vi "MIU_Control_v1.4 - Working - has bugs still.vi"() -> ()   [LabVIEW 2010]
uses:
  <vilib>/Utility/error.llb/DialogType.ctl
  <vilib>/Instr/_visa.llb/VISA Configure Serial Port (Instr).vi
  <vilib>/Analysis/NI_AALPro.lvlib
panel:
  in  "Tab Control":T1(tab)
  in  "Serial Read Port":refnum<visa-resource-name>="COM5"
  in  "data bits":u16=8 min=5 max=8 step=1
  in  "parity":u16(ring) items=["None", "Odd", "Even", "Mark", "Space"]
  in  "stop bits":u16(ring)=10 items=["1.0"=10, "1.5"=15, "2.0"=20]
  in  "flow control":u16(ring) items=["None"=0, "XON/XOFF"=1, "RTS/CTS"=2, "DTR/DSR"=4]
  in  "delay before read (ms)":u32=500
  in  "byte count":u32=500
  out "Incoming Serial String":string="    02/28/13 05:18:49.492,    3.20644e-01,    0.00000e+00,    3.33105e-01,    0.00000e+00,    5.19723e+02,    0.00000e+00,    3.20811e-01,    0.00000e+00,    3.33278e-01,    0.00000e+00,    8.02680e+01,    0.00000e+00,    3.33389e+01,    0.00000e+00,    2.71783e+01,    0.00000e+00,    3.55973e-01,    0.00000e+00,    6.31022e-01,    0.00000e+00,    1.95007e+00,    0.00000e+00,              3\n"
  out "Time":string="05:18:49.492"
  out "Date":string="02/28/13"
  out "return count":u32=394
  in  "Instrument baud rate (9600)":u32=9600
  in  "Control Port":refnum<visa-resource-name>="COM4"
  in  "Control baud rate":u32=9600
  out "N2O is FLAT":bool
  out "Rolling CO Slope Fit":cluster{i32[], "Best Linear Fit":dbl[]}[](graph)=[{[0, 1, 2, 3, 4, 5, 6, 7, 8, 9, 10, 11, 12, 13, 14, 15, 16, 17, 18, 19], "Best Linear Fit"=[0.320611, 0.320505, 0.320476, 0.3208, 0.320926, 0.320701, 0.320587, 0.320889, 0.320914, 0.320439, 0.3209, 0.320794, 0.320847, 0.320592, 0.320735, 0.32085, 0.320821, 0.320729, 0.320589, 0.320309]}, {[0, 1, 2, 3, 4, 5, 6, 7, 8, 9, 10, 11, 12, 13, 14, 15, 16, 17, 18, 19], "Best Linear Fit"=[0.32070674285714285, 0.3207061067669173, 0.3207054706766917, 0.32070483458646615, 0.3207041984962406, 0.32070356240601505, 0.32070292631578945, 0.3207022902255639, 0.32070165413533835, 0.3207010180451128, 0.3207003819548872, 0.32069974586466166, 0.3206991097744361, 0.32069847368421056, 0.32069783759398496, 0.3206972015037594, 0.32069656541353386, 0.32069592932330826, 0.3206952932330827, 0.32069465714285716]}]
  out "CO":dbl(graph)=0.320644
  out "N2O":dbl(graph)=0.333105
  out "H2O":dbl(graph)=519.723
  out "CO PPM":string=" 3.20644e-01"
  out "N2O PPM":string="3.33105e-01"
  out "H2O PPM":string="5.19723e+02"
  in  "Points to Average":i32=30
  out "CO Slope":dbl=-6.360902255623756e-07
  out "Rolling N2O Slope Fit 2":cluster{i32[], "Best Linear Fit":dbl[]}[](graph)=[{[0, 1, 2, 3, 4, 5, 6, 7, 8, 9, 10, 11, 12, 13, 14, 15, 16, 17, 18, 19], "Best Linear Fit"=[0.333232, 0.332975, 0.333256, 0.333094, 0.333062, 0.3332, 0.332763, 0.333281, 0.333155, 0.333115, 0.333375, 0.33321, 0.333348, 0.33294, 0.333468, 0.333464, 0.333003, 0.333373, 0.33336, 0.333239]}, {[0, 1, 2, 3, 4, 5, 6, 7, 8, 9, 10, 11, 12, 13, 14, 15, 16, 17, 18, 19], "Best Linear Fit"=[0.33308077142857145, 0.33309286390977444, 0.3331049563909775, 0.33311704887218047, 0.3331291413533835, 0.3331412338345865, 0.3331533263157895, 0.3331654187969925, 0.3331775112781955, 0.33318960375939854, 0.33320169624060153, 0.3332137887218045, 0.33322588120300756, 0.33323797368421054, 0.3332500661654135, 0.33326215864661657, 0.33327425112781955, 0.3332863436090226, 0.3332984360902256, 0.33331052857142857]}]
  out "N2O Slope":dbl=1.209248120300707e-05
  in  "N2O Low Limit":dbl=-1e-05
  in  "CO High Limit":dbl=1e-05
  out "CO is FLAT":bool
  in  "CO Low Limit":dbl=-1e-05
  in  "N2O High Limit":dbl=1e-05
  out "Switch Valve":bool
  out "Boolean":bool
  in  "Manually Switch Valves":bool=TRUE
  in  "Valve to switch":dbl=1.0 min=0.0 max=16.0 step=1.0
  in  "stop":bool
  in  "Switching Delay (s)":dbl=60.0
  out "Current Valve":dbl=1.0
  in  "Number of Bottles":dbl=5.0
  out "CELL TEMP":string="3.33389e+01"
  out "CELL TEMPERATURE":dbl(graph)=33.3389
  out "AMBIENT TEMPERATURE":dbl(graph)=27.1783
  out "AMBIENT TEMP":string="2.71783e+01"
  out "AIN5":dbl(graph)=0.631022
  out "SUPERCOOL TEMP":string="6.31022e-01"
  out "LINE LOCK":dbl(graph)=0.355973
  out "LINELOCK - LASER CONTROL VOLTAGE":string="3.55973e-01"
  out "PRESSURE":dbl(graph)=80.268
  out "PRESSURE 2":string="8.02680e+01"
  out "CO DRY 2":dbl(graph)=0.320811
  out "N2O DRY":dbl(graph)=0.333278
  out "CO DRY":string="3.20811e-01"
  out "N2O DRY 2":string="3.33278e-01"
  # "Automatic Linearization"
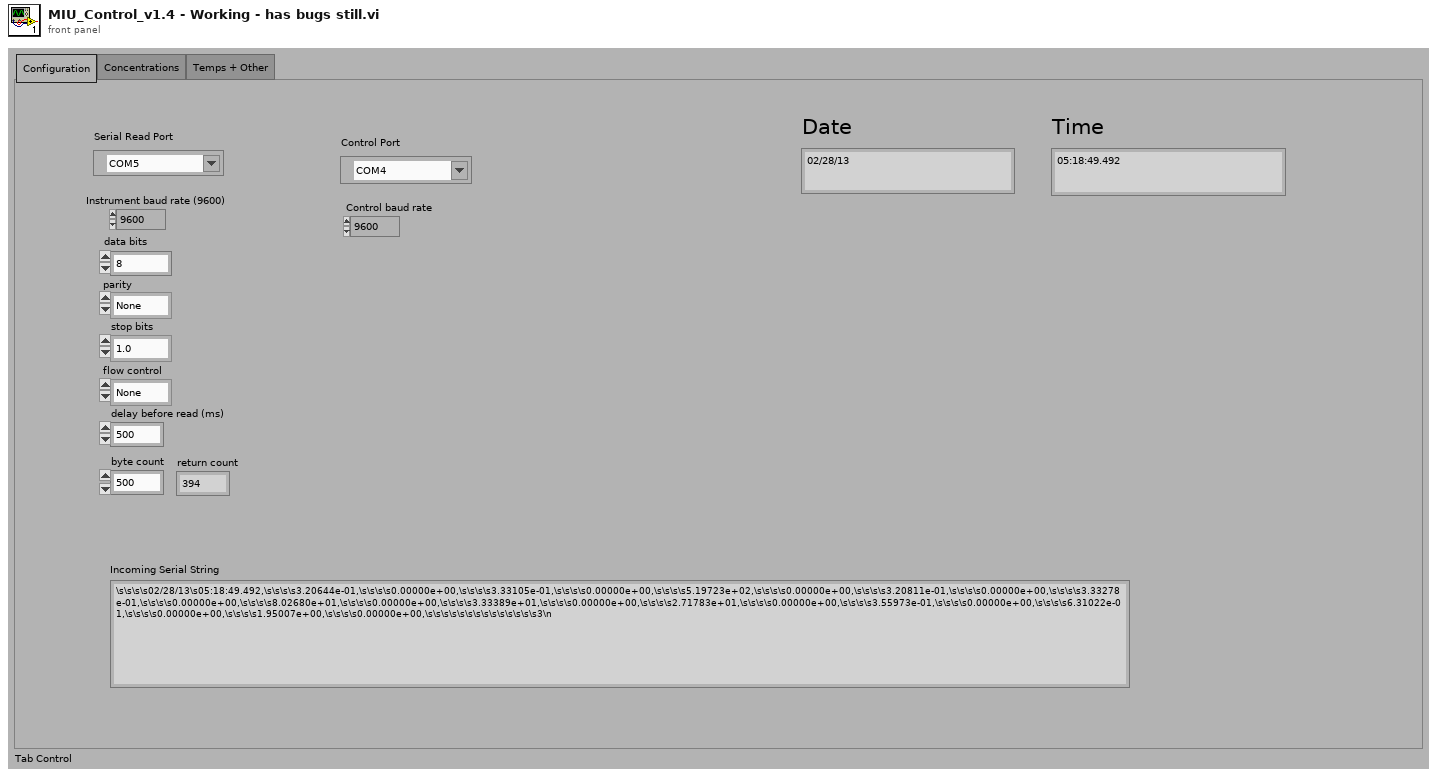
[diagram p1: front panel]
types:
  T1 = enum32{"Configuration", "Concentrations", "Temps + Other"}
  T2 = typedef "DialogType.ctl" = u16
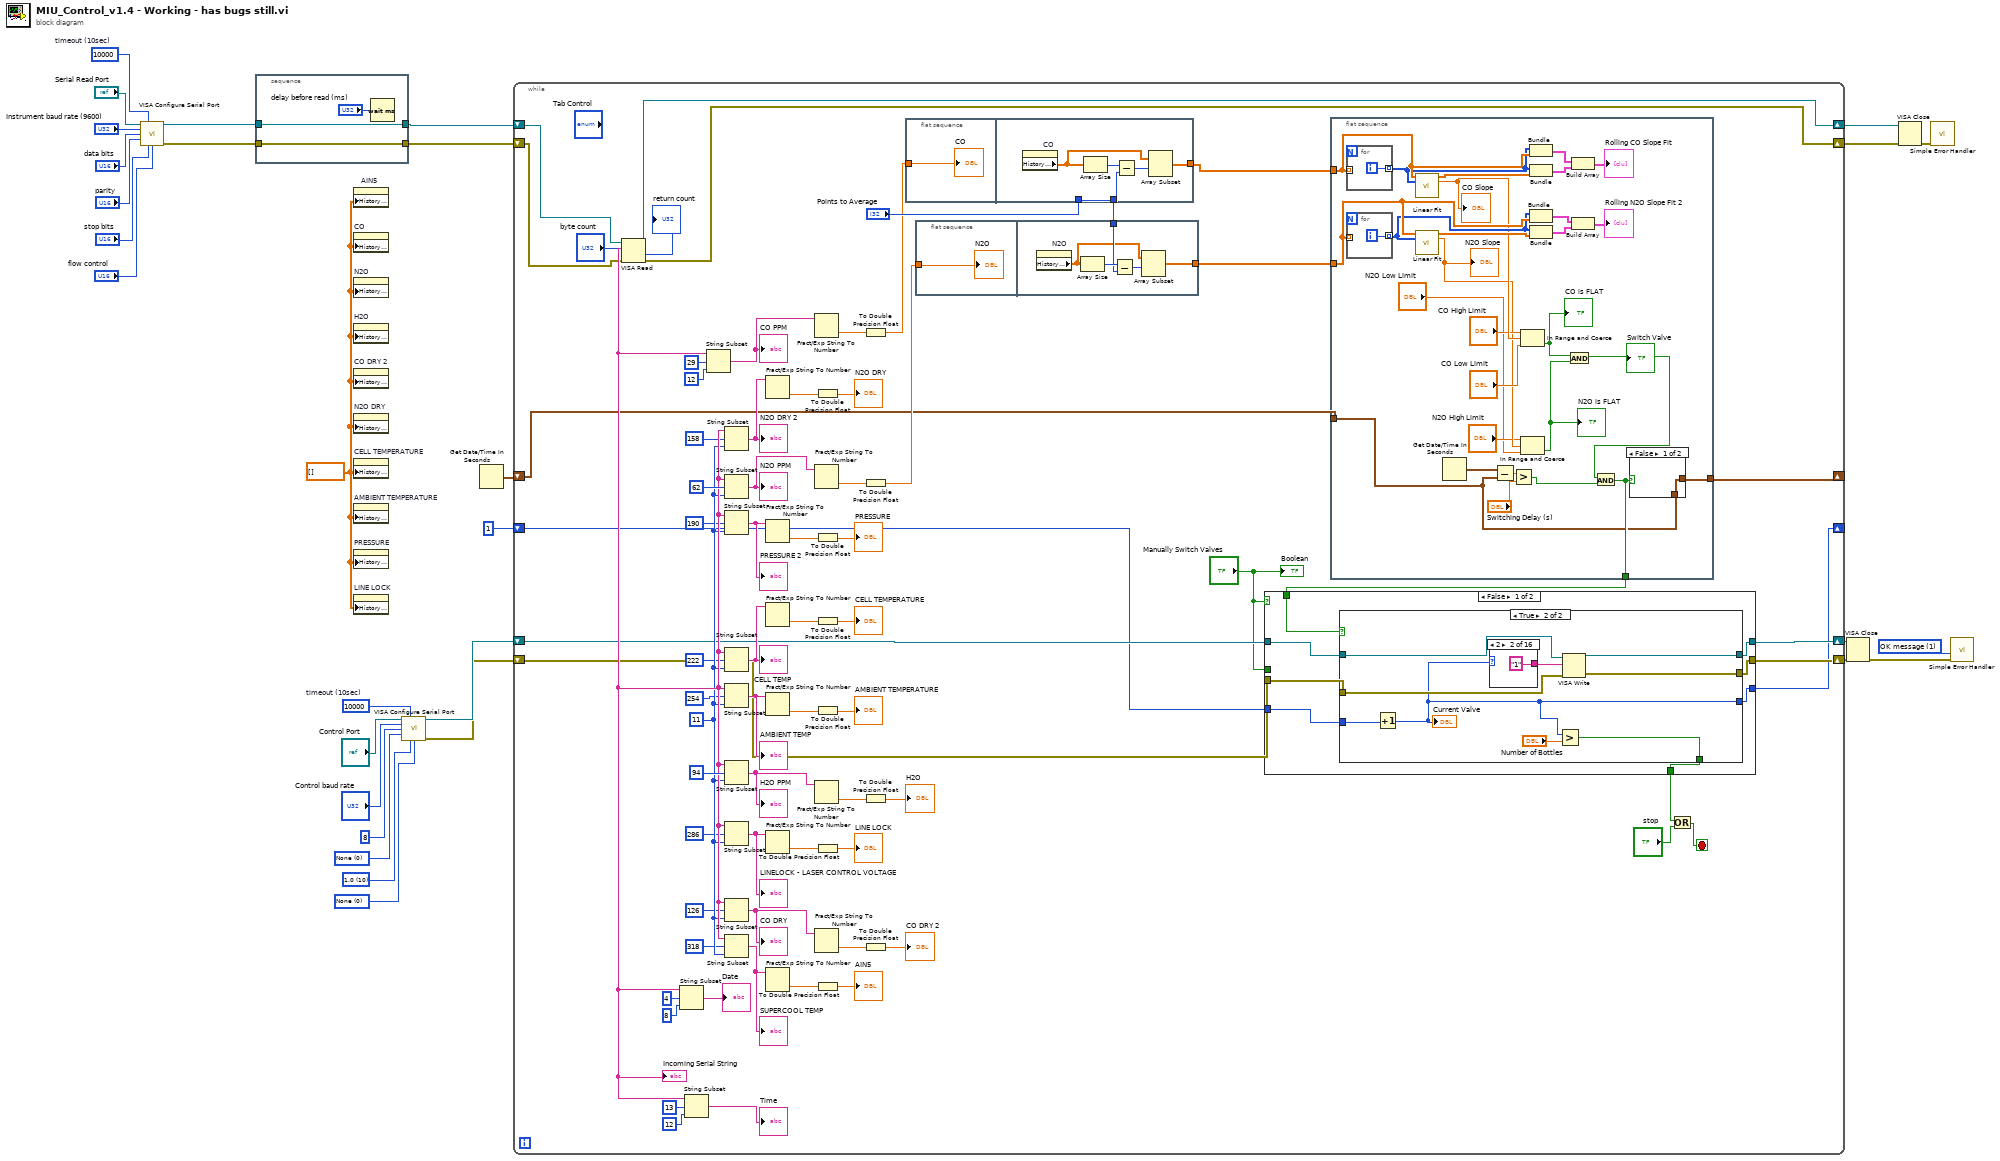
[diagram p0: block diagram]
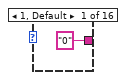
[diagram p3: hidden frame]
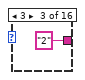
[diagram p4: hidden frame]
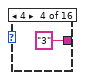
[diagram p5: hidden frame]
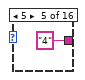
[diagram p6: hidden frame]
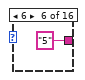
[diagram p7: hidden frame]
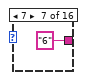
[diagram p8: hidden frame]
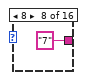
[diagram p9: hidden frame]
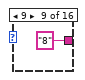
[diagram p10: hidden frame]
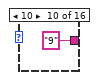
[diagram p11: hidden frame]
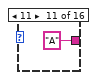
[diagram p12: hidden frame]
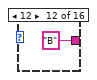
[diagram p13: hidden frame]
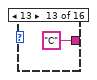
[diagram p14: hidden frame]
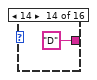
[diagram p15: hidden frame]
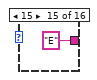
[diagram p16: hidden frame]
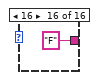
[diagram p17: hidden frame]
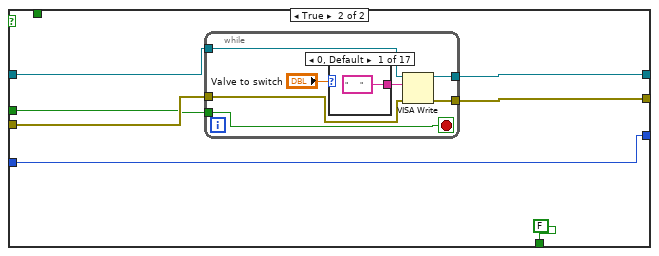
[diagram p18: hidden frame]
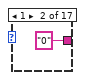
[diagram p19: hidden frame]
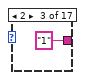
[diagram p20: hidden frame]
diagram:
  w9 = T2 1 items=["no dialog", "OK message", "continue or stop message", "OK message + warnings", "continue/stop + warnings"] ("type of dialog (OK msg:1)")
  w13 = u16 0 items=["None"=0, "XON/XOFF"=1, "RTS/CTS"=2, "DTR/DSR"=4] ("flow control")
  w14 = u16 10 items=["1.0"=10, "1.5"=15, "2.0"=20] ("stop bits")
  w16 = u16 0 items=["None", "Odd", "Even", "Mark", "Space"] ("parity")
  w15 = u32 10000  # timeout (10sec)
  w19 = dbl[] [] ("History Data")
  w27 = u32 10000  # timeout (10sec)
  n1 = call-poly "VISA Configure Serial Port"("VISA resource name"="Serial Read Port", "timeout (10sec)"=w27, "baud rate (9600)"="Instrument baud rate (9600)", "data bits (8)"="data bits", "parity (0:none)"="parity", "stop bits (10: 1 bit)"="stop bits", "flow control (0:none)"="flow control") -> ("VISA resource name out"=w22:refnum<visa-resource-name>, "error out"=w23:errorcluster)  [unwired: 2 in, 5 out]
  n2 = stacked-sequence {
    tunnel: w23 -> [w33]
    tunnel: [w33] -> w1
    tunnel: w22 -> [w32]
    tunnel: [w32] -> w2
    frame #0 {
      n3 = Wait (ms)(milliseconds to wait="delay before read (ms)") -> ()  [unwired: 1 out]
    }
  }
  n4 = property on="AIN5" class="WFChart (strict)"("History Data"=w19) -> ()  [unwired: 2 in, 2 out]
  n5 = property on="CO" class="WFChart (strict)"("History Data"=w19) -> ()  [unwired: 2 in, 2 out]
  n6 = property on="N2O" class="WFChart (strict)"("History Data"=w19) -> ()  [unwired: 2 in, 2 out]
  n7 = property on="H2O" class="WFChart (strict)"("History Data"=w19) -> ()  [unwired: 2 in, 2 out]
  n8 = property on="CO DRY 2" class="WFChart (strict)"("History Data"=w19) -> ()  [unwired: 2 in, 2 out]
  n9 = property on="N2O DRY" class="WFChart (strict)"("History Data"=w19) -> ()  [unwired: 2 in, 2 out]
  n10 = property on="CELL TEMPERATURE" class="WFChart (strict)"("History Data"=w19) -> ()  [unwired: 2 in, 2 out]
  n11 = property on="AMBIENT TEMPERATURE" class="WFChart (strict)"("History Data"=w19) -> ()  [unwired: 2 in, 2 out]
  n12 = property on="PRESSURE" class="WFChart (strict)"("History Data"=w19) -> ()  [unwired: 2 in, 2 out]
  n13 = property on="LINE LOCK" class="WFChart (strict)"("History Data"=w19) -> ()  [unwired: 2 in, 2 out]
  n14 = call-poly "VISA Configure Serial Port"("VISA resource name"="Control Port", "timeout (10sec)"=w15, "baud rate (9600)"="Control baud rate", "data bits (8)"=u16 8 ("data bits"), "parity (0:none)"=w16, "stop bits (10: 1 bit)"=w14, "flow control (0:none)"=w13) -> ("VISA resource name out"=w8:refnum<visa-resource-name>, "error out"=w7:errorcluster)  [unwired: 2 in, 5 out]
  n15 = Get Date/Time In Seconds() -> (seconds since 1Jan1904=w3:timestamp)
  n16 = while {
    shift-right: [w50] -> w6
    shift-left: w8 -> [w48]
    shift-right: [w49] -> w5
    shift-left: w7 -> [w47]
    shift-right: [w99] -> w21
    shift-left: w2 -> [w41]
    shift-right: [w58] -> w20
    shift-left: w1 -> [w42]
    shift-right: [w39] -> _
    shift-left: 1 -> [w40]
    shift-right: [w36] -> _
    shift-left: w3 -> [w38]
    stop <- w53 stop-if-true
    w68 = 11 ("offset (0)")
    n17 = VISA Read(VISA resource name=w41, byte count="byte count", error in (no error)=w42) -> (VISA resource name out=w99:refnum<visa-resource-name>, read buffer=w69:string, return count=→"return count":u32, error out=w58:errorcluster)
    "Incoming Serial String" <- w69
    n18 = String Subset(string=w69, offset (0)=4, length (rest)=8 ("length (rest)")) -> (substring=→"Date":string)
    n19 = String Subset(string=w69, offset (0)=13, length (rest)=12 ("length (rest)")) -> (substring=→"Time":string)
    n20 = String Subset(string=w69, offset (0)=29, length (rest)=12 ("length (rest)")) -> (substring=w94:string)
    "CO PPM" <- w94
    n21 = String Subset(string=w69, offset (0)=158, length (rest)=w68) -> (substring=w80:string)
    "N2O DRY 2" <- w80
    n22 = String Subset(string=w69, offset (0)=62, length (rest)=w68) -> (substring=w93:string)
    "N2O PPM" <- w93
    n23 = String Subset(string=w69, offset (0)=190, length (rest)=w68) -> (substring=w79:string)
    "PRESSURE 2" <- w79
    n24 = String Subset(string=w69, offset (0)=222, length (rest)=w68) -> (substring=w78:string)
    "CELL TEMP" <- w78
    n25 = String Subset(string=w69, offset (0)=254, length (rest)=w68) -> (substring=w72:string)
    "AMBIENT TEMP" <- w72
    n26 = String Subset(string=w69, offset (0)=94, length (rest)=w68) -> (substring=w92:string)
    "H2O PPM" <- w92
    n27 = String Subset(string=w69, offset (0)=286, length (rest)=w68) -> (substring=w71:string)
    "LINELOCK - LASER CONTROL VOLTAGE" <- w71
    n28 = String Subset(string=w69, offset (0)=126, length (rest)=w68) -> (substring=w81:string)
    "CO DRY" <- w81
    n29 = String Subset(string=w69, offset (0)=318, length (rest)=w68) -> (substring=w70:string)
    "SUPERCOOL TEMP" <- w70
    n30 = Fract/Exp String To Number(string=w80) -> (number=w86:dbl)  [unwired: 3 in, 1 out]
    n31 = Fract/Exp String To Number(string=w79) -> (number=w84:dbl)  [unwired: 3 in, 1 out]
    n32 = Fract/Exp String To Number(string=w78) -> (number=w82:dbl)  [unwired: 3 in, 1 out]
    n33 = Fract/Exp String To Number(string=w72) -> (number=w76:dbl)  [unwired: 3 in, 1 out]
    n34 = Fract/Exp String To Number(string=w71) -> (number=w74:dbl)  [unwired: 3 in, 1 out]
    n35 = Fract/Exp String To Number(string=w70) -> (number=w73:dbl)  [unwired: 3 in, 1 out]
    n36 = Fract/Exp String To Number(string=w94) -> (number=w91:dbl)  [unwired: 3 in, 1 out]
    n37 = Fract/Exp String To Number(string=w93) -> (number=w57:dbl)  [unwired: 3 in, 1 out]
    n38 = Fract/Exp String To Number(string=w92) -> (number=w90:dbl)  [unwired: 3 in, 1 out]
    n39 = Fract/Exp String To Number(string=w81) -> (number=w88:dbl)  [unwired: 3 in, 1 out]
    n40 = To Double Precision Float(number=w86) -> (double precision float=→"N2O DRY":dbl)
    n41 = To Double Precision Float(number=w84) -> (double precision float=→"PRESSURE":dbl)
    n42 = To Double Precision Float(number=w82) -> (double precision float=→"CELL TEMPERATURE":dbl)
    n43 = To Double Precision Float(number=w76) -> (double precision float=→"AMBIENT TEMPERATURE":dbl)
    n44 = To Double Precision Float(number=w74) -> (double precision float=→"LINE LOCK":dbl)
    n45 = To Double Precision Float(number=w73) -> (double precision float=→"AIN5":dbl)
    n46 = To Double Precision Float(number=w91) -> (double precision float=w52:dbl)
    n47 = To Double Precision Float(number=w57) -> (double precision float=w51:dbl)
    n48 = To Double Precision Float(number=w90) -> (double precision float=→"H2O":dbl)
    n49 = To Double Precision Float(number=w88) -> (double precision float=→"CO DRY 2":dbl)
    n50 = flat-sequence {
      tunnel: w52 -> [w212]
      tunnel: [w214] -> w44
      tunnel: "Points to Average" -> [w213]
      tunnel: [w213] -> w55
      frame #0 {
        "CO" <- w212
      }
      frame #1 {
        n51 = property on="CO" class="WFChart (strict)"() -> ("History Data"=w215:dbl[])  [unwired: 2 in, 2 out]
        n52 = Array Size(array=w215) -> (size(s)=w216:i32)
        n53 = Subtract(x=w216, y=w213) -> (x-y=w217:i32)
        n54 = Array Subset(array=w215, index=w217) -> (w214:dbl[])  [unwired: 1 in]
      }
    }
    n55 = flat-sequence {
      tunnel: w51 -> [w206]
      tunnel: w55 -> [w209]
      tunnel: [w207] -> w45
      frame #0 {
        "N2O" <- w206
      }
      frame #1 {
        n56 = property on="N2O" class="WFChart (strict)"() -> ("History Data"=w208:dbl[])  [unwired: 2 in, 2 out]
        n57 = Array Size(array=w208) -> (size(s)=w210:i32)
        n58 = Subtract(x=w210, y=w209) -> (x-y=w211:i32)
        n59 = Array Subset "Array Subset"(array=w208, index=w211) -> (w207:dbl[])  [unwired: 1 in]
      }
    }
    n60 = case shown="False" "Manually Switch Valves" {
      tunnel: [w113 w149] -> w50
      tunnel: [w112 w148] -> w49
      tunnel: w48 -> [w111 w147]
      tunnel: w47 -> [w110 w146]
      tunnel: "Manually Switch Valves" -> [_ w145]
      tunnel: [w109 FALSE] -> w35
      tunnel: w40 -> [w108 w143]
      tunnel: w37 -> [w107 _]
      tunnel: [w106 w143] -> w39
      frame False {
        n61 = case shown="True" w107 {
          selector: w107 -> [w115 _]
          tunnel: [w117 w124] -> w113
          tunnel: [w116 w125] -> w112
          tunnel: w111 -> [w117 w123]
          tunnel: w110 -> [w116 w122]
          tunnel: [w115 w120] -> w109
          tunnel: w108 -> [w114 w119]
          tunnel: [w114 w118] -> w106
          frame False {
          }
          frame True {
            n62 = Increment(x=w119) -> (x+1=w118:i32)
            "Current Valve" <- w118
            n63 = case shown="2" w118 {
              tunnel: ["0" "1" "2" "3" "4" "5" "6" "7" "8" "9" "A" "B" "C" "D" "E" "F"] -> w126
              frame 1, Default {
              }
              frame 2 {
              }
              frame 3 {
              }
              frame 4 {
              }
              frame 5 {
              }
              frame 6 {
              }
              frame 7 {
              }
              frame 8 {
              }
              frame 9 {
              }
              frame 10 {
              }
              frame 11 {
              }
              frame 12 {
              }
              frame 13 {
              }
              frame 14 {
              }
              frame 15 {
              }
              frame 16 {
              }
            }
            n64 = Greater?(x=w118, y="Number of Bottles") -> (0:w120:bool)
            n65 = VISA Write(VISA resource name=w123, write buffer=w126, error in (no error)=w122) -> (VISA resource name out=w124:refnum<visa-resource-name>, error out=w125:errorcluster)  [unwired: 1 out]
          }
        }
      }
      frame True {
        n66 = while {
          tunnel: [w154] -> w149
          tunnel: [w153] -> w148
          tunnel: w147 -> [w152]
          tunnel: w146 -> [w151]
          tunnel: w145 -> [w150]
          stop <- w150 stop-if-true
          n67 = case shown="0, Default" "Valve to switch" {
            tunnel: ["      " "0" "1" "2" "3" "4" "5" "6" "7" "8" "9" "A" "B" "C" "D" "E" "F"] -> w156
            frame 0, Default {
            }
            frame 1 {
            }
            frame 2 {
            }
            frame 3 {
            }
            frame 4 {
            }
            frame 5 {
            }
            frame 6 {
            }
            frame 7 {
            }
            frame 8 {
            }
            frame 9 {
            }
            frame 10 {
            }
            frame 11 {
            }
            frame 12 {
            }
            frame 13 {
            }
            frame 14 {
            }
            frame 15 {
            }
            frame 16 {
            }
          }
          n68 = VISA Write(VISA resource name=w152, write buffer=w156, error in (no error)=w151) -> (VISA resource name out=w154:refnum<visa-resource-name>, error out=w153:errorcluster)  [unwired: 1 out]
        }
      }
    }
    n69 = flat-sequence {
      tunnel: w44 -> [w201]
      tunnel: w45 -> [w200]
      tunnel: w38 -> [w174]
      tunnel: [w176] -> w37
      tunnel: [w175] -> w36
      frame #0 {
        n70 = for {
          tunnel: [w205] -> w199 mode=indexing
          tunnel: w201 -> [_] mode=indexing
          i -> [w205]
        }
        n71 = for {
          tunnel: [w204] -> w194 mode=indexing
          tunnel: w200 -> [_] mode=indexing
          i -> [w204]
        }
        n72 = call <vilib>:"Linear Fit.vi"("Y"=w201, "X"=w199) -> ("Best Linear Fit"=w198:dbl[], "slope"=w189:dbl)  [unwired: 9 in, 3 out]
        "CO Slope" <- w189
        n73 = call <vilib>:"Linear Fit.vi"("Y"=w200, "X"=w194) -> ("Best Linear Fit"=w193:dbl[], "slope"=w186:dbl)  [unwired: 9 in, 3 out]
        "N2O Slope" <- w186
        n74 = Get Date/Time In Seconds() -> (seconds since 1Jan1904=w181:timestamp)
        n75 = Subtract(x=w181, y=w174) -> (x-y=w180:dbl)
        n76 = Greater?(x=w180, y="Switching Delay (s)") -> (0:w178:bool)
        n77 = In Range and Coerce(upper limit="CO High Limit", x=w189, lower limit="CO Low Limit") -> (In Range?=w183:bool)  [unwired: 1 out]
        "CO is FLAT" <- w183
        n78 = In Range and Coerce(upper limit="N2O High Limit", x=w186, lower limit="N2O Low Limit") -> (In Range?=w182:bool)  [unwired: 1 out]
        "N2O is FLAT" <- w182
        n79 = Bundle(w199, w201) -> (w197:cluster{i32[], dbl[]})  [unwired: 1 in]
        n80 = Bundle(w199, "Best Linear Fit"=w198) -> (w196:cluster{i32[], "Best Linear Fit":dbl[]})  [unwired: 1 in]
        n81 = Bundle(w194, w200) -> (w192:cluster{i32[], dbl[]})  [unwired: 1 in]
        n82 = Bundle(w194, "Best Linear Fit"=w193) -> (w191:cluster{i32[], "Best Linear Fit":dbl[]})  [unwired: 1 in]
        n83 = And(x=w183, y=w182) -> (x .and. y?=w177:bool)
        "Switch Valve" <- w177
        n84 = Build Array(w197, w196) -> (→"Rolling CO Slope Fit":cluster{i32[], "Best Linear Fit":dbl[]}[])
        n85 = Build Array(w192, w191) -> (→"Rolling N2O Slope Fit 2":cluster{i32[], "Best Linear Fit":dbl[]}[])
        n86 = And(x=w177, y=w178) -> (x .and. y?=w176:bool)
        n87 = case shown="False" w176 {
          tunnel: [w202 w203] -> w175
          tunnel: w174 -> [w202 _]
          frame False {
          }
          frame True {
            n88 = Get Date/Time In Seconds() -> (seconds since 1Jan1904=w203:timestamp)
          }
        }
      }
    }
    n89 = Or(x=w35, y="stop") -> (x .or. y?=w53:bool)
    "Boolean" <- "Manually Switch Valves"
  }
  n90 = VISA Close(VISA resource name=w6, error in (no error)=w5) -> (error out=w11:errorcluster)
  n91 = VISA Close(VISA resource name=w21, error in (no error)=w20) -> (error out=w29:errorcluster)
  n92 = call <vilib>:"Simple Error Handler.vi"("error in (no error)"=w29) -> ()  [unwired: 1 in, 8 out]
  n93 = call <vilib>:"Simple Error Handler.vi"("type of dialog (OK msg:1)"=w9, "error in (no error)"=w11) -> ()  [unwired: 8 out]
